vi "limitswitchcontroll.vi"(9 "Up Switch":bool, 10 "Numeric":dbl, 11 "Down Switch":bool) -> (3 "t":dbl)   [LabVIEW 2011]
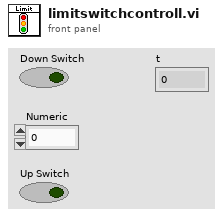
[diagram p1: front panel]
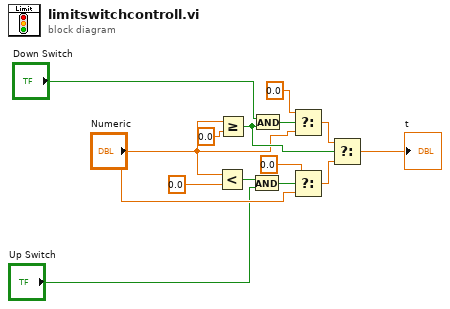
[diagram p0: block diagram]
diagram:
  n1 = Less?(x="Numeric", y=0.0) -> (x < y?=w3:bool)
  n2 = Greater Or Equal?(x="Numeric", y=0.0) -> (x >= y?=w13:bool)
  n3 = And(x=w3, y="Up Switch") -> (x .and. y?=w5:bool)
  n4 = And(x="Down Switch", y=w13) -> (x .and. y?=w8:bool)
  n5 = Select(t=0.0, s=w8, f="Numeric") -> (s? t:f=w11:dbl)
  n6 = Select(t=0.0, s=w5, f="Numeric") -> (s? t:f=w12:dbl)
  n7 = Select(t=w11, s=w13, f=w12) -> (s? t:f=→"t":dbl)
